vi "CAN_LIN_Demo_Template.vi"() -> ()   [LabVIEW 2014]
uses:
  TSMaster_API/All_Control/Typedef/Hardware Type.ctl
  Utilities/Typedef/Hardware_Subtype.ctl
  TSMaster_API/LIN_Function/Typedef/TSLIN_SetData.ctl
  TSMaster_API/LIN_Function/Typedef/TSLIN_Transmit.ctl
  TSMaster_API/CAN_CANFD_Function/Typedef/TSCAN_CANFD_Configuration.ctl
  TSMaster_API/CAN_CANFD_Function/Typedef/TLibCANFD.ctl
  TSMaster_API/LIN_Function/Typedef/TLibLIN.ctl
panel:
  out "ACANMsgBuffer":T1(array[cluster])
  out "ALINBuffer":T2[](array[typedef])
  # "使用方法：\n1.创建TSMaster 工程，映射CAN/LIN通道2，并开启接收Trace\n2.此demo 映射通道1\n3.通道1与通道2进行短接\n4.运行此demo 发送Fdata ,并接收Fdata"
  # "usage method:\n1. Create TSMaster project, map CAN/LIN channel 2, and enable receiving Trace. \n2. This demo maps channel 1. \n3. Short circuit channel 1 to channel 2\n4. Run this demo sends and receives Fdata"
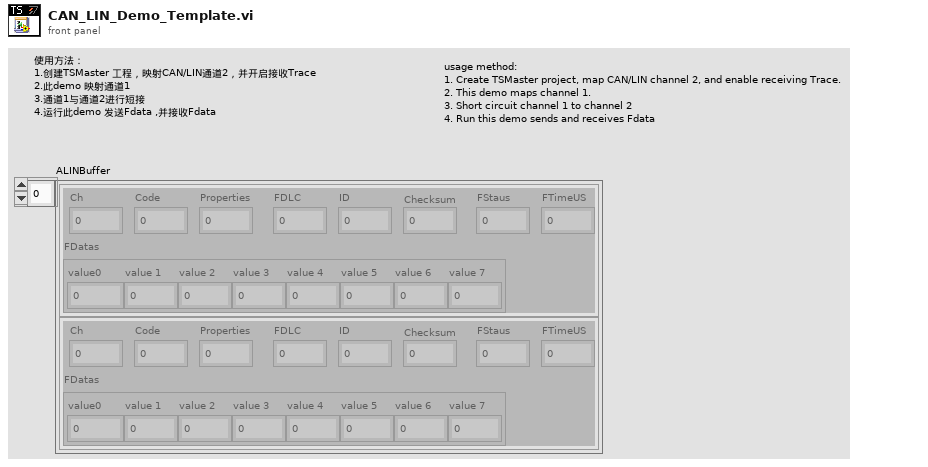
[diagram p1: front panel]
types:
  T1 = cluster{"FIdxChn":u8, "FProperties":u8, "FDLC":u8, "FReserved":u8, "FIdentifier":i32, "FTimeUS":u64, "Fdata":cluster{"初始化的数组[0]":u8, "初始化的数组[1]":u8, "初始化的数组[2]":u8, "初始化的数组[3]":u8, "初始化的数组[4]":u8, "初始化的数组[5]":u8, "初始化的数组[6]":u8, "初始化的数组[7]":u8, "初始化的数组[8]":u8, "初始化的数组[9]":u8, "初始化的数组[10]":u8, "初始化的数组[11]":u8, "初始化的数组[12]":u8, "初始化的数组[13]":u8, "初始化的数组[14]":u8, "初始化的数组[15]":u8, "初始化的数组[16]":u8, "初始化的数组[17]":u8, "初始化的数组[18]":u8, "初始化的数组[19]":u8, "初始化的数组[20]":u8, "初始化的数组[21]":u8, "初始化的数组[22]":u8, "初始化的数组[23]":u8, "初始化的数组[24]":u8, "初始化的数组[25]":u8, "初始化的数组[26]":u8, "初始化的数组[27]":u8, "初始化的数组[28]":u8, "初始化的数组[29]":u8, "初始化的数组[30]":u8, "初始化的数组[31]":u8, "初始化的数组[32]":u8, "初始化的数组[33]":u8, "初始化的数组[34]":u8, "初始化的数组[35]":u8, "初始化的数组[36]":u8, "初始化的数组[37]":u8, "初始化的数组[38]":u8, "初始化的数组[39]":u8, "初始化的数组[40]":u8, "初始化的数组[41]":u8, "初始化的数组[42]":u8, "初始化的数组[43]":u8, "初始化的数组[44]":u8, "初始化的数组[45]":u8, "初始化的数组[46]":u8, "初始化的数组[47]":u8, "初始化的数组[48]":u8, "初始化的数组[49]":u8, "初始化的数组[50]":u8, "初始化的数组[51]":u8, "初始化的数组[52]":u8, "初始化的数组[53]":u8, "初始化的数组[54]":u8, "初始化的数组[55]":u8, "初始化的数组[56]":u8, "初始化的数组[57]":u8, "初始化的数组[58]":u8, "初始化的数组[59]":u8, "初始化的数组[60]":u8, "初始化的数组[61]":u8, "初始化的数组[62]":u8, "初始化的数组[63]":u8}}[]
  T2 = typedef "TLibLIN.ctl" = cluster{"Ch":u8, "Code":u8, "Properties":u8, "FDLC":u8, "ID":u8, "Checksum":u8, "FStaus":u8, "FTimeUS":u64, "FDatas":cluster{"value0":u8, "value 1":u8, "value 2":u8, "value 3":u8, "value 4":u8, "value 5":u8, "value 6":u8, "value 7":u8}}
  T3 = typedef "TSCAN_CANFD_Configuration.ctl" = cluster{"Hardware Type":T4, "Hardware Subtype":T5, "AArbRateKbps":sgl, "AListenOnly":enum16{"Normal", "ListenOnly"}, "Int120Ohm":enum16{"Disable", "Enable"}, "EnableChannel":enum16{"Disable", "Enable"}, "AHwChannel":i32, "AAppChannel":i32, "ADataRateKbps":sgl, "AControllerType":i32, "AControllerMode":i32, "AldHW":i32}
  T4 = typedef "Hardware Type.ctl" = i32
  T5 = typedef "Hardware_Subtype.ctl" = enum16{"TS_UNKNOWN_DEVICE", "TSCAN_PRO", "TSCAN_Lite1", "TC1001", "TL1001", "TC1011", "TM5011", "TC1002", "TC1014", "TSCANFD2517", "TC1026", "TC1016", "TC1012", "TC1013", "TLog1002", "TC1034", "TC1018", "GW2116", "TC2115", "MP1013", "TC1113", "TC1114", "TP1013", "TC1017", "TP1018", "TF10XX", "TL1004_FD_4_LIN_2", "TE1051", "TP1051", "TP1034", "TTS9015", "TP1026", "TTS1026", "TTS1034", "TTS1018", "TL1011", "TTS1015_LiAuto", "TTS1013_LiAuto", "TTS1016Pro", "TC1054Pro", "TC1054", "TLog1038", "TO1013", "TC1034Pro", "TC1018Pro", "TC1038Pro", "TS_DEV_END"}
  T6 = enum16{"Only read received messages", "Receive&send messages"}
  T7 = typedef "TSLIN_SetData.ctl" = cluster{"Hardware Type":T4, "Hardware Subtype":T5, "AHwChannel":i32, "AAppChannel":i32, "ABaudrateKbps":sgl, "AProtocol":i32, "AldHW":i32}
  T8 = typedef "TLibCANFD.ctl" = cluster{"AIdxchn":u8, "AId":i32, "AIsStd":u8, "BRS":enum16{"Close", "Open"}, "AIsData":u8, "ADLC":i32, "AIsFD":enum16{"Classic CAN Message", "FD CAN Message"}, "FDatas":cluster{"Initialize array[0]":u8, "Initialize array[1]":u8, "Initialize array[2]":u8, "Initialize array[3]":u8, "Initialize array[4]":u8, "Initialize array[5]":u8, "Initialize array[6]":u8, "Initialize array[7]":u8, "Initialize array[8]":u8, "Initialize array[9]":u8, "Initialize array[10]":u8, "Initialize array[11]":u8, "Initialize array[12]":u8, "Initialize array[13]":u8, "Initialize array[14]":u8, "Initialize array[15]":u8, "Initialize array[16]":u8, "Initialize array[17]":u8, "Initialize array[18]":u8, "Initialize array[19]":u8, "Initialize array[20]":u8, "Initialize array[21]":u8, "Initialize array[22]":u8, "Initialize array[23]":u8, "Initialize array[24]":u8, "Initialize array[25]":u8, "Initialize array[26]":u8, "Initialize array[27]":u8, "Initialize array[28]":u8, "Initialize array[29]":u8, "Initialize array[30]":u8, "Initialize array[31]":u8, "Initialize array[32]":u8, "Initialize array[33]":u8, "Initialize array[34]":u8, "Initialize array[35]":u8, "Initialize array[36]":u8, "Initialize array[37]":u8, "Initialize array[38]":u8, "Initialize array[39]":u8, "Initialize array[40]":u8, "Initialize array[41]":u8, "Initialize array[42]":u8, "Initialize array[43]":u8, "Initialize array[44]":u8, "Initialize array[45]":u8, "Initialize array[46]":u8, "Initialize array[47]":u8, "Initialize array[48]":u8, "Initialize array[49]":u8, "Initialize array[50]":u8, "Initialize array[51]":u8, "Initialize array[52]":u8, "Initialize array[53]":u8, "Initialize array[54]":u8, "Initialize array[55]":u8, "Initialize array[56]":u8, "Initialize array[57]":u8, "Initialize array[58]":u8, "Initialize array[59]":u8, "Initialize array[60]":u8, "Initialize array[61]":u8, "Initialize array[62]":u8, "Initialize array[63]":u8}}
  T9 = typedef "TSLIN_Transmit.ctl" = cluster{"Channel":i32, "Rx/TX":enum16{"Rx", "Tx"}, "Set_node_funtiontype":i32, "DLC":u32, "ID":u32, "FDatas":cluster{"value0":u8, "value 1":u8, "value 2":u8, "value 3":u8, "value 4":u8, "value 5":u8, "value 6":u8, "value 7":u8}}
  T10 = cluster{"数组[0]":u8, "数组[1]":u8, "数组[2]":u8, "数组[3]":u8, "数组[4]":u8, "数组[5]":u8, "数组[6]":u8, "数组[7]":u8, "数组[8]":u8, "数组[9]":u8, "数组[10]":u8, "数组[11]":u8, "数组[12]":u8, "数组[13]":u8, "数组[14]":u8, "数组[15]":u8, "数组[16]":u8, "数组[17]":u8, "数组[18]":u8, "数组[19]":u8, "数组[20]":u8, "数组[21]":u8, "数组[22]":u8, "数组[23]":u8, "数组[24]":u8, "数组[25]":u8, "数组[26]":u8, "数组[27]":u8, "数组[28]":u8, "数组[29]":u8, "数组[30]":u8, "数组[31]":u8, "数组[32]":u8, "数组[33]":u8, "数组[34]":u8, "数组[35]":u8, "数组[36]":u8, "数组[37]":u8, "数组[38]":u8, "数组[39]":u8, "数组[40]":u8, "数组[41]":u8, "数组[42]":u8, "数组[43]":u8, "数组[44]":u8, "数组[45]":u8, "数组[46]":u8, "数组[47]":u8, "数组[48]":u8, "数组[49]":u8, "数组[50]":u8, "数组[51]":u8, "数组[52]":u8, "数组[53]":u8, "数组[54]":u8, "数组[55]":u8, "数组[56]":u8, "数组[57]":u8, "数组[58]":u8, "数组[59]":u8, "数组[60]":u8, "数组[61]":u8, "数组[62]":u8, "数组[63]":u8}
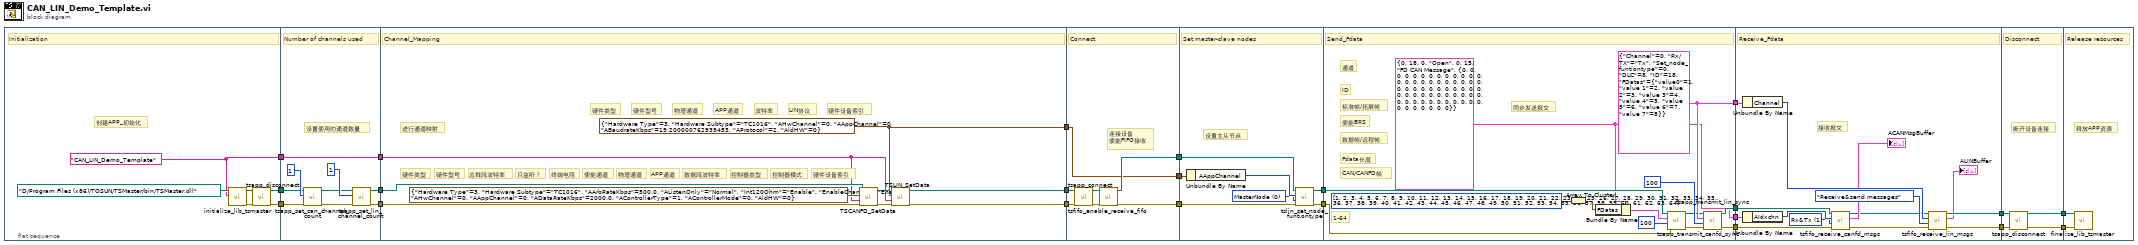
[diagram p0: block diagram]
diagram:
  n1 = flat-sequence {
    tunnel: [w25] -> w22
    tunnel: [w24] -> w21
    tunnel: [w23] -> w17
    tunnel: w22 -> [w30]
    tunnel: w21 -> [w32]
    tunnel: [w36] -> w20
    tunnel: [w35] -> w19
    tunnel: [w34] -> w18
    tunnel: w17 -> [w34]
    tunnel: w20 -> [w42]
    tunnel: w19 -> [w41]
    tunnel: w18 -> [w38]
    tunnel: [w46] -> w16
    tunnel: [w45] -> w15
    tunnel: [w44] -> w12
    tunnel: w16 -> [w52]
    tunnel: w15 -> [w50]
    tunnel: [w49] -> w14
    tunnel: [w48] -> w13
    tunnel: w12 -> [w47]
    tunnel: [w47] -> w11
    tunnel: w14 -> [w60]
    tunnel: w13 -> [w59]
    tunnel: w11 -> [w58]
    tunnel: [w55] -> w10
    tunnel: [w54] -> w9
    tunnel: w10 -> [w65]
    tunnel: w9 -> [w64]
    tunnel: [w72] -> w8
    tunnel: [w71] -> w7
    tunnel: [w70] -> w6
    tunnel: [w61] -> w1
    tunnel: w8 -> [w77]
    tunnel: w7 -> [w76]
    tunnel: w6 -> [w87]
    tunnel: [w84] -> w5
    tunnel: [w83] -> w4
    tunnel: w1 -> [w78]
    tunnel: w5 -> [w91]
    tunnel: w4 -> [w90]
    tunnel: [w89] -> w3
    tunnel: [w88] -> w2
    tunnel: w3 -> [w93]
    tunnel: w2 -> [w92]
    frame #0 {
      w23 = "CAN_LIN_Demo_Template" ("AppName")
      # "创建APP_初始化"
      # "Initialization"
      n2 = call "initialize_lib_tsmaster.vi"("AppName"=w23, "Path input"=path "D:/Program Files (x86)/TOSUN/TSMaster/bin/TSMaster.dll") -> ("error output"=w28:errorcluster, "Path output"=w27:path)  [unwired: 8 in]
      n3 = call "tsapp_disconnect.vi"("error in (no error)"=w28, "Path"=w27) -> ("error output"=w24:errorcluster, "Path output"=w25:path)  [unwired: 7 in, 1 out]
    }
    frame #1 {
      # "设置使用的通道数量"
      # "Number of channels used"
      n4 = call "tsapp_set_can_channel_count.vi"("error in (no error)"=w32, "Aount"=1, "Path"=w30) -> ("error out"=w31:errorcluster, "Path output"=w29:path)  [unwired: 6 in, 1 out]
      n5 = call "tsapp_set_lin_channel_count.vi"("error in (no error)"=w31, "Aount"=1, "Path"=w29) -> ("error out"=w35:errorcluster, "Path output"=w36:path)  [unwired: 6 in, 1 out]
    }
    frame #2 {
      w44 = T7 {"Hardware Type"=3, "Hardware Subtype"=enum."TC1016", "AHwChannel"=0, "AAppChannel"=0, "ABaudrateKbps"=19.2, "AProtocol"=2, "AldHW"=0} ("Set")
      # "硬件设备索引"
      # "LIN协议"
      # "波特率"
      # "APP通道"
      # "物理通道"
      # "硬件型号"
      # "硬件类型"
      # "硬件设备索引"
      # "控制器模式"
      # "控制器类型"
      # "数据段波特率"
      # "APP通道"
      # "物理通道"
      # "使能通道"
      # "终端电阻"
      # "只监听？"
      # "总裁段波特率"
      # "硬件型号"
      # "硬件类型"
      # "进行通道映射"
      # "Channel_Mapping"
      n6 = call "TSCANFD_SetData.vi"("ERROR IN"=w41, "AppName"=w38, "CANFD Configuration"=T3 {"Hardware Type"=3, "Hardware Subtype"=enum."TC1016", "AArbRateKbps"=500.0, "AListenOnly"=enum."Normal", "Int120Ohm"=enum."Enable", "EnableChannel"=enum."Enable", "AHwChannel"=0, "AAppChannel"=0, "ADataRateKbps"=2000.0, "AControllerType"=1, "AControllerMode"=0, "AldHW"=0}, "PATH"=w42) -> ("ERROR OUT"=w39:errorcluster, "PATH OUT"=w40:path)  [unwired: 4 in, 2 out]
      n7 = call "TSLIN_SetData.vi"("Error in"=w39, "AppName"=w38, "Set"=w44, "Path"=w40) -> ("Error out"=w45:errorcluster, "Path output"=w46:path)  [unwired: 4 in, 2 out]
    }
    frame #3 {
      # "连接设备\n使能FIFO接收"
      # "Connect"
      n8 = call "tsapp_connect.vi"("error in (no error)"=w50, "Path"=w52) -> ("error out"=w53:errorcluster, "Path output"=w51:path)  [unwired: 7 in, 1 out]
      n9 = call "tsfifo_enable_receive_fifo.vi"("error in (no error)"=w53, "Path"=w51) -> ("error out"=w48:errorcluster, "Path output"=w49:path)  [unwired: 8 in]
    }
    frame #4 {
      w56 = 0 items=["MasterNode", "SlaveNode", "MonitorNote"] ("set_node_funtiontype")
      # "设置主从节点"
      # "Set master-slave nodes"
      n10 = Unbundle By Name(w58) -> ("AAppChannel"=w57:i32)
      n11 = call "tslin_set_node_funtiontype.vi"("错误输入（无错误）"=w59, "set_node_funtiontype"=w56, "AAppChannel"=w57, "path"=w60) -> ("错误输出"=w54:errorcluster, "path out"=w55:path)  [unwired: 5 in, 1 out]
    }
    frame #5 {
      w61 = T8 {"AIdxchn"=0, "AId"=18, "AIsStd"=0, "BRS"=enum."Open", "AIsData"=0, "ADLC"=15, "AIsFD"=enum."FD CAN Message", "FDatas"={"Initialize array[0]"=0, "Initialize array[1]"=0, "Initialize array[2]"=0, "Initialize array[3]"=0, "Initialize array[4]"=0, "Initialize array[5]"=0, "Initialize array[6]"=0, "Initialize array[7]"=0, "Initialize array[8]"=0, "Initialize array[9]"=0, "Initialize array[10]"=0, "Initialize array[11]"=0, "Initialize array[12]"=0, "Initialize array[13]"=0, "Initialize array[14]"=0, "Initialize array[15]"=0, "Initialize array[16]"=0, "Initialize array[17]"=0, "Initialize array[18]"=0, "Initialize array[19]"=0, "Initialize array[20]"=0, "Initialize array[21]"=0, "Initialize array[22]"=0, "Initialize array[23]"=0, "Initialize array[24]"=0, "Initialize array[25]"=0, "Initialize array[26]"=0, "Initialize array[27]"=0, "Initialize array[28]"=0, "Initialize array[29]"=0, "Initialize array[30]"=0, "Initialize array[31]"=0, "Initialize array[32]"=0, "Initialize array[33]"=0, "Initialize array[34]"=0, "Initialize array[35]"=0, "Initialize array[36]"=0, "Initialize array[37]"=0, "Initialize array[38]"=0, "Initialize array[39]"=0, "Initialize array[40]"=0, "Initialize array[41]"=0, "Initialize array[42]"=0, "Initialize array[43]"=0, "Initialize array[44]"=0, "Initialize array[45]"=0, "Initialize array[46]"=0, "Initialize array[47]"=0, "Initialize array[48]"=0, "Initialize array[49]"=0, "Initialize array[50]"=0, "Initialize array[51]"=0, "Initialize array[52]"=0, "Initialize array[53]"=0, "Initialize array[54]"=0, "Initialize array[55]"=0, "Initialize array[56]"=0, "Initialize array[57]"=0, "Initialize array[58]"=0, "Initialize array[59]"=0, "Initialize array[60]"=0, "Initialize array[61]"=0, "Initialize array[62]"=0, "Initialize array[63]"=0}} ("TCANFD")
      w70 = T9 {"Channel"=0, "Rx/TX"=enum."Tx", "Set_node_funtiontype"=0, "DLC"=8, "ID"=18, "FDatas"={"value0"=1, "value 1"=2, "value 2"=3, "value 3"=4, "value 4"=5, "value 5"=6, "value 6"=7, "value 7"=8}} ("LIN_Transmit")
      # "CAN/CANFD帧"
      # "Fdata长度"
      # "数据帧/远程帧"
      # "使能BRS"
      # "标准帧/拓展帧"
      # "ID"
      # "通道"
      # "1-64"
      # "同步发送报文"
      # "Send_Fdata"
      n12 = Array To Cluster(array=u8[] [1, 2, 3, 4, 5, 6, 7, 8, 9, 10, 11, 12, 13, 14, 15, 16, 17, 18, 19, 20, 21, 22, 23, 24, 25, 26, 27, 28, 29, 30, 31, 32, 33, 34, 35, 36, 37, 38, 39, 40, 41, 42, 43, 44, 45, 46, 47, 48, 49, 50, 51, 52, 53, 54, 55, 56, 57, 58, 59, 60, 61, 62, 63, 64] ("数组")) -> (cluster=w68:T10)
      n13 = Bundle By Name(cluster=w61, "FDatas"=w68) -> (w67:T8)
      n14 = call "tsapp_transmit_canfd_sync.vi"("error in (no error)"=w64, "ATimeoutMS"=100, "TCANFD"=w67, "Path"=w65) -> ("error out"=w62:errorcluster, "Path output"=w63:path)  [unwired: 5 in, 1 out]
      n15 = call "tsapp_transmit_lin_sync.vi"("错误输入（无错误）"=w62, "ATimeoutMS"=100, "LIN_Transmit"=w70, "路径输入"=w63) -> ("错误输出"=w71:errorcluster, "路径输出"=w72:path)  [unwired: 5 in, 1 out]
    }
    frame #6 {
      w80 = u16 1 items=["Rx", "Rx&Tx"] ("Display message type")
      # "接收报文"
      # "Receive_Fdata"
      n16 = Unbundle By Name(w87) -> ("Channel"=w86:i32)
      n17 = Unbundle By Name(w78) -> ("AIdxchn"=w81:u8)
      n18 = call "tsfifo_receive_canfd_msgs.vi"("error in (no error)"=w76, "Display message type"=w80, "AAPPChannel"=w81, "Path"=w77) -> ("error out"=w74:errorcluster, "ACANMsgBuffer"=→"ACANMsgBuffer":T1, "Path output"=w75:path)  [unwired: 3 in, 1 out]
      n19 = call "tsfifo_receive_lin_msgs.vi"("错误输入（无错误）"=w74, "Read message type"=T6."Receive&send messages", "AIdxChn"=w86, "路径输入"=w75) -> ("错误输出"=w83:errorcluster, "ALINBuffer"=→"ALINBuffer":T2[], "路径输出"=w84:path)  [unwired: 4 in, 1 out]
    }
    frame #7 {
      # "断开设备连接"
      # "Disconnect"
      n20 = call "tsapp_disconnect.vi"("error in (no error)"=w90, "Path"=w91) -> ("error output"=w89:errorcluster, "Path output"=w88:path)  [unwired: 7 in, 1 out]
    }
    frame #8 {
      # "释放APP资源"
      # "Release resources"
      n21 = call "finalize_lib_tsmaster.vi"("error in (no error)"=w93, "Path"=w92) -> ()  [unwired: 8 in, 2 out]
    }
  }
